vi "RSxxx Protocol FG.vi"(7 "Action":T1, 8 "error in (no error)":errorcluster, 10 "Serial Config":T2={"Port"="COM1", "Baud Rate"=9600, "Data Bits"=8, "Parity"=enum."None", "Stop Bits"=10, "Flow Control"=0, "XON"=enum."DC1", "XOFF"=enum."DC3", "End Read on Termination Character"=TRUE, "End Write on Termination Character"=TRUE, "Termination Character"=10} {"Termination Character" format="%.0x"; "Flow Control" items=["None"=0, "XON/XOFF"=1, "RTS/CTS"=2, "DTR/DSR"=4]; "Stop Bits" items=["1.0"=10, "1.5"=15, "2.0"=20]; "Data Bits" min=5 max=8 step=1; "Baud Rate" items=["75"=75, "110"=110, "134"=134, "150"=150, "300"=300, "600"=600, "1200"=1200, "1800"=1800, "2400"=2400, "4800"=4800, "7200"=7200, "9600"=9600, "14400"=14400, "19200"=19200, "28800"=28800, "38400"=38400, "56000"=56000, "57600"=57600, "115200"=115200, "128000"=128000, "230400"=230400, "460800"=460800, "921600"=921600, "1843200"=1843200, "3000000"=3000000]}, 11 "Device Item Ref in":T3 format="%.0x") -> (0 "error out":errorcluster, 2 "Serial Config":T2 {"Termination Character" format="%.0x"; "Flow Control" items=["None"=0, "XON/XOFF"=1, "RTS/CTS"=2, "DTR/DSR"=4]; "Stop Bits" items=["1.0"=10, "1.5"=15, "2.0"=20]; "Data Bits" min=5 max=8 step=1; "Baud Rate" items=["75"=75, "110"=110, "134"=134, "150"=150, "300"=300, "600"=600, "1200"=1200, "1800"=1800, "2400"=2400, "4800"=4800, "7200"=7200, "9600"=9600, "14400"=14400, "19200"=19200, "28800"=28800, "38400"=38400, "56000"=56000, "57600"=57600, "115200"=115200, "128000"=128000, "230400"=230400, "460800"=460800, "921600"=921600, "1843200"=1843200, "3000000"=3000000]}, 3 "Item Ref out":T3 format="%.0x")   [LabVIEW 2018, in "Instrument Addon Shared.lvlib"]
uses:
  Instrument Addon Shared.lvlib
  <vilib>/NI Veristand/Custom Device API/Custom Device Item Ref.ctl
  Types/RSXXX Port Settings.ctl
  Types/FG Control.ctl
  Constants.vi
  <vilib>/NI Veristand/Custom Device API/Get Item Property (String).vi
  <vilib>/NI Veristand/Custom Device API/Get Item Property (U32).vi
  <vilib>/NI Veristand/Custom Device API/Get Item Property (Boolean).vi
  <vilib>/NI Veristand/Custom Device API/Set Item Property (String).vi
  <vilib>/NI Veristand/Custom Device API/Set Item Property (U32).vi
  <vilib>/NI Veristand/Custom Device API/Set Item Property (Boolean).vi
  <vilib>/NI Veristand/Custom Device API/Custom Device API.lvlib
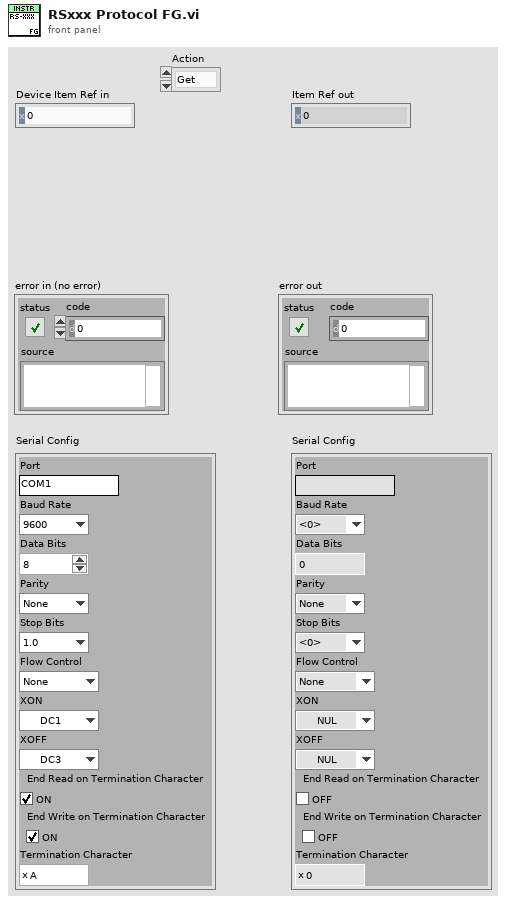
[diagram p1: front panel]
types:
  T1 = typedef "Instrument Addon Shared.lvlib/FG Control.ctl" = enum16{"Get", "Set"}
  T2 = typedef "Instrument Addon Shared.lvlib/RSXXX Port Settings.ctl" = cluster{"Port":string, "Baud Rate":u32, "Data Bits":u16, "Parity":enum16{"None", "Odd", "Even", "Mark", "Space"}, "Stop Bits":u16, "Flow Control":u16, "XON":enum16{"NUL", "SOH", "STX", "ETX", "EOT", "ENQ", "ACK", "BEL", "BS", "HT", "LF", "VT", "FF", "CR", "SO", "SI", "DLE", "DC1", "DC2", "DC3", "DC4", "NAK", "SYN", "ETB", "CAN", "EM", "SUB", "ESC", "FS", "GS", "RS", "US", "SP", "!", "\"", "#", "$", "%", "&", "'", "(", ")", "*", "+", ",", "- (-)", ".", "/", "0", "1", "2", "3", "4", "5", "6", "7", "8", "9", ":", ";", "<", "=", ">", "?", "@", "A", "B", "C", "D", "E", "F", "G", "H", "I", "J", "K", "L", "M", "N", "O", "P", "Q", "R", "S", "T", "U", "V", "W", "X", "Y", "Z", "[", "\\", "]", "^", "_", "`", "a", "b", "c", "d", "e", "f", "g", "h", "i", "j", "k", "l", "m", "n", "o", "p", "q", "r", "s", "t", "u", "v", "w", "x", "y", "z", "{", "|", "}", "~"}, "XOFF":enum16{"NUL", "SOH", "STX", "ETX", "EOT", "ENQ", "ACK", "BEL", "BS", "HT", "LF", "VT", "FF", "CR", "SO", "SI", "DLE", "DC1", "DC2", "DC3", "DC4", "NAK", "SYN", "ETB", "CAN", "EM", "SUB", "ESC", "FS", "GS", "RS", "US", "SP", "!", "\"", "#", "$", "%", "&", "'", "(", ")", "*", "+", ",", "- (-)", ".", "/", "0", "1", "2", "3", "4", "5", "6", "7", "8", "9", ":", ";", "<", "=", ">", "?", "@", "A", "B", "C", "D", "E", "F", "G", "H", "I", "J", "K", "L", "M", "N", "O", "P", "Q", "R", "S", "T", "U", "V", "W", "X", "Y", "Z", "[", "\\", "]", "^", "_", "`", "a", "b", "c", "d", "e", "f", "g", "h", "i", "j", "k", "l", "m", "n", "o", "p", "q", "r", "s", "t", "u", "v", "w", "x", "y", "z", "{", "|", "}", "~"}, "End Read on Termination Character":bool, "End Write on Termination Character":bool, "Termination Character":u8}
  T3 = typedef "Custom Device API.lvlib/Custom Device Item Ref.ctl" = u64
  T4 = enum16{"NUL", "SOH", "STX", "ETX", "EOT", "ENQ", "ACK", "BEL", "BS", "HT", "LF", "VT", "FF", "CR", "SO", "SI", "DLE", "DC1", "DC2", "DC3", "DC4", "NAK", "SYN", "ETB", "CAN", "EM", "SUB", "ESC", "FS", "GS", "RS", "US", "SP", "!", "\"", "#", "$", "%", "&", "'", "(", ")", "*", "+", ",", "- (-)", ".", "/", "0", "1", "2", "3", "4", "5", "6", "7", "8", "9", ":", ";", "<", "=", ">", "?", "@", "A", "B", "C", "D", "E", "F", "G", "H", "I", "J", "K", "L", "M", "N", "O", "P", "Q", "R", "S", "T", "U", "V", "W", "X", "Y", "Z", "[", "\\", "]", "^", "_", "`", "a", "b", "c", "d", "e", "f", "g", "h", "i", "j", "k", "l", "m", "n", "o", "p", "q", "r", "s", "t", "u", "v", "w", "x", "y", "z", "{", "|", "}", "~"}
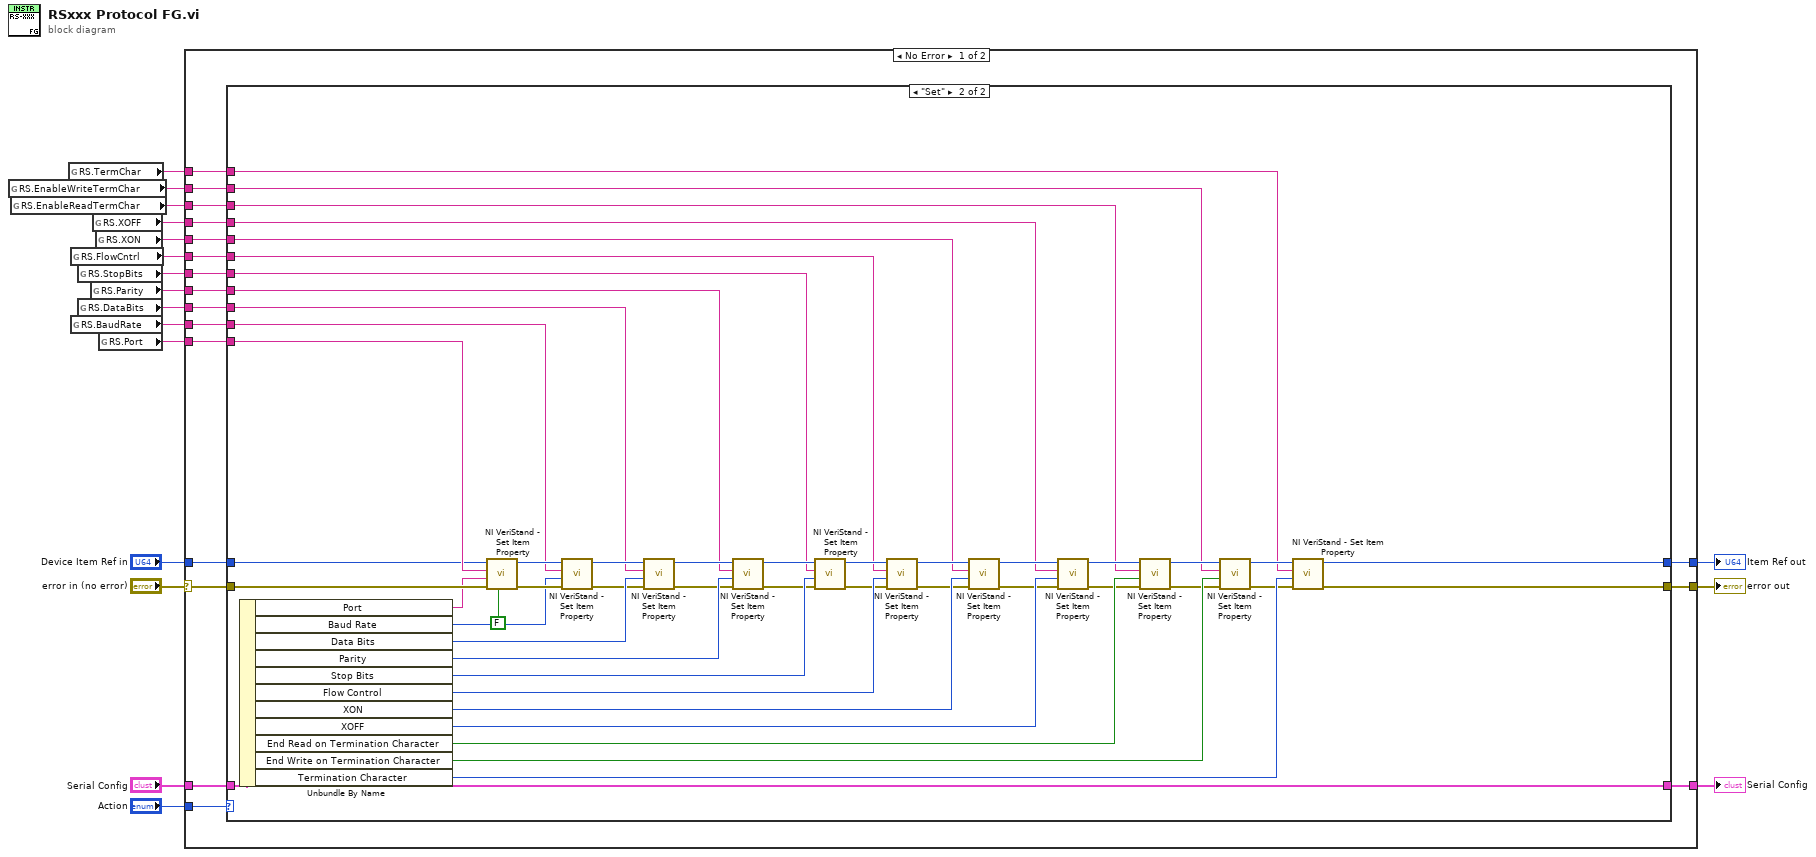
[diagram p0: block diagram]
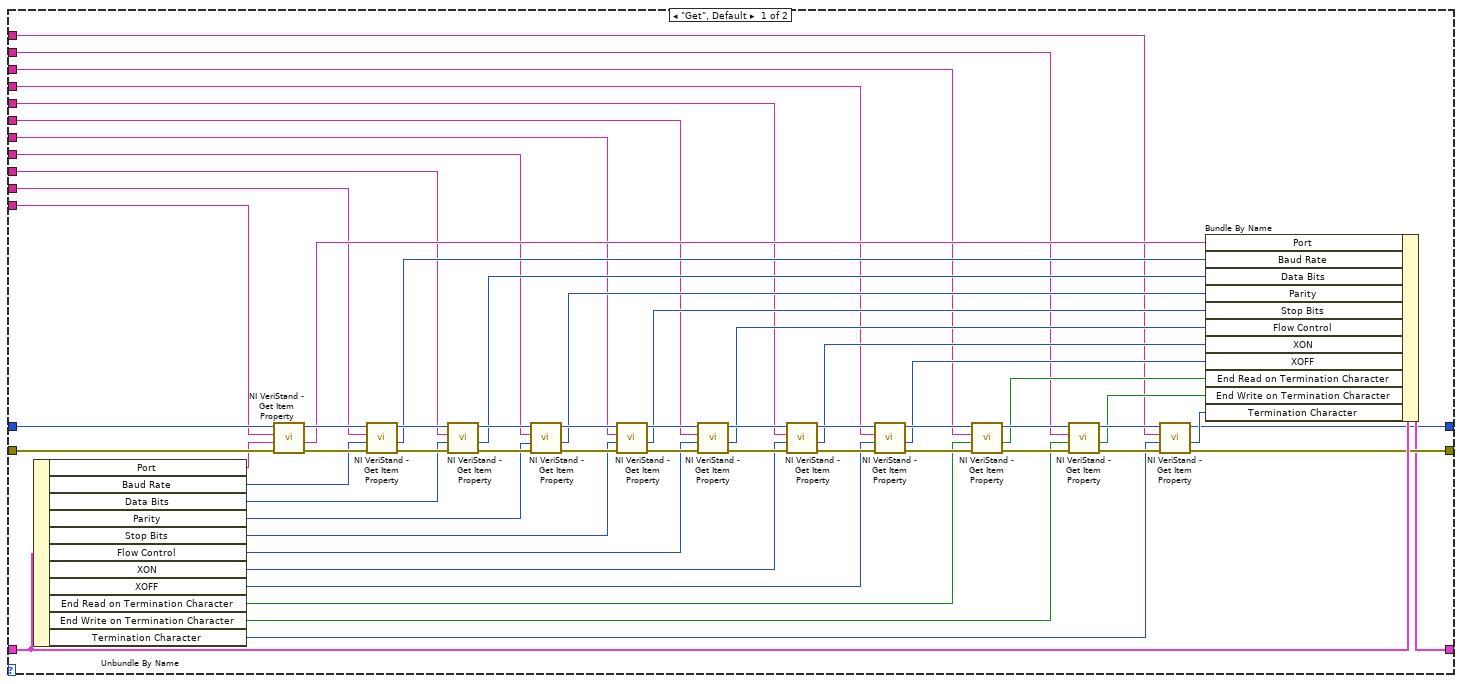
[diagram p2: hidden frame]
diagram:
  n1 = global read "Constants.vi" "RS.EnableWriteTermChar"() -> (w2:string)
  n2 = global read "Constants.vi" "RS.EnableReadTermChar"() -> (w3:string)
  n3 = global read "Constants.vi" "RS.TermChar"() -> (w1:string)
  n4 = global read "Constants.vi" "RS.FlowCntrl"() -> (w6:string)
  n5 = global read "Constants.vi" "RS.BaudRate"() -> (w10:string)
  n6 = global read "Constants.vi" "RS.StopBits"() -> (w7:string)
  n7 = global read "Constants.vi" "RS.DataBits"() -> (w9:string)
  n8 = global read "Constants.vi" "RS.Parity"() -> (w8:string)
  n9 = global read "Constants.vi" "RS.XOFF"() -> (w4:string)
  n10 = global read "Constants.vi" "RS.XON"() -> (w5:string)
  n11 = global read "Constants.vi" "RS.Port"() -> (w18:string)
  n12 = case shown="No Error" "error in (no error)" {
    selector: "error in (no error)" -> [w31 w146]
    tunnel: w18 -> [w36 _]
    tunnel: [w35 w144] -> w17
    tunnel: "Device Item Ref in" -> [w34 w144]
    tunnel: "Serial Config" -> [w33 w145]
    tunnel: [w32 w146] -> w14
    tunnel: [w30 w145] -> w12
    tunnel: "Action" -> [w29 _]
    tunnel: w10 -> [w28 _]
    tunnel: w9 -> [w27 _]
    tunnel: w8 -> [w26 _]
    tunnel: w7 -> [w25 _]
    tunnel: w6 -> [w24 _]
    tunnel: w5 -> [w23 _]
    tunnel: w4 -> [w22 _]
    tunnel: w3 -> [w21 _]
    tunnel: w2 -> [w20 _]
    tunnel: w1 -> [w19 _]
    frame No Error {
      n13 = case shown="\"Set\"" w29 {
        tunnel: w36 -> [w93 w143]
        tunnel: [w47 w106] -> w35
        tunnel: w34 -> [w94 w142]
        tunnel: w33 -> [w61 w140]
        tunnel: [w49 w107] -> w32
        tunnel: w31 -> [w95 w141]
        tunnel: [w48 w140] -> w30
        tunnel: w28 -> [w46 w105]
        tunnel: w27 -> [w45 w104]
        tunnel: w26 -> [w44 w103]
        tunnel: w25 -> [w43 w102]
        tunnel: w24 -> [w42 w101]
        tunnel: w23 -> [w41 w100]
        tunnel: w22 -> [w40 w99]
        tunnel: w21 -> [w39 w98]
        tunnel: w20 -> [w38 w97]
        tunnel: w19 -> [w37 w96]
        frame "Get", Default {
          n14 = Unbundle By Name(w61) -> ("Port"=w92:string, "Baud Rate"=w71:u32, "Data Bits"=w70:u16, "Parity"=w69:enum16{"None", "Odd", "Even", "Mark", "Space"}, "Stop Bits"=w68:u16, "Flow Control"=w67:u16, "XON"=w66:T4, "XOFF"=w65:T4, "End Read on Termination Character"=w64:bool, "End Write on Termination Character"=w63:bool, "Termination Character"=w62:u8)
          n15 = call-poly <vilib>:"NI VeriStand - Get Item Property.vi"("error in (no error)"=w95, "Default Value"=w92, "Property Name"=w93, "Item Ref in"=w94) -> ("error out"=w81:errorcluster, "Value"=w60:string, "Item Ref out"=w91:T3)  [unwired: 4 in, 1 out]
          n16 = call-poly <vilib>:"NI VeriStand - Get Item Property.vi"("error in (no error)"=w81, "Default Value"=w71, "Property Name"=w46, "Item Ref in"=w91) -> ("error out"=w80:errorcluster, "Value"=w59:u32, "Item Ref out"=w90:T3)  [unwired: 4 in, 1 out]
          n17 = call-poly <vilib>:"NI VeriStand - Get Item Property.vi"("error in (no error)"=w80, "Default Value"=w70, "Property Name"=w45, "Item Ref in"=w90) -> ("error out"=w79:errorcluster, "Value"=w58:u32, "Item Ref out"=w89:T3)  [unwired: 4 in, 1 out]
          n18 = call-poly <vilib>:"NI VeriStand - Get Item Property.vi"("error in (no error)"=w79, "Default Value"=w69, "Property Name"=w44, "Item Ref in"=w89) -> ("error out"=w78:errorcluster, "Value"=w57:u32, "Item Ref out"=w88:T3)  [unwired: 4 in, 1 out]
          n19 = call-poly <vilib>:"NI VeriStand - Get Item Property.vi"("error in (no error)"=w78, "Default Value"=w68, "Property Name"=w43, "Item Ref in"=w88) -> ("error out"=w77:errorcluster, "Value"=w56:u32, "Item Ref out"=w87:T3)  [unwired: 4 in, 1 out]
          n20 = call-poly <vilib>:"NI VeriStand - Get Item Property.vi"("error in (no error)"=w77, "Default Value"=w67, "Property Name"=w42, "Item Ref in"=w87) -> ("error out"=w76:errorcluster, "Value"=w55:u32, "Item Ref out"=w86:T3)  [unwired: 4 in, 1 out]
          n21 = call-poly <vilib>:"NI VeriStand - Get Item Property.vi"("error in (no error)"=w76, "Default Value"=w66, "Property Name"=w41, "Item Ref in"=w86) -> ("error out"=w75:errorcluster, "Value"=w54:u32, "Item Ref out"=w85:T3)  [unwired: 4 in, 1 out]
          n22 = call-poly <vilib>:"NI VeriStand - Get Item Property.vi"("error in (no error)"=w75, "Default Value"=w65, "Property Name"=w40, "Item Ref in"=w85) -> ("error out"=w74:errorcluster, "Value"=w53:u32, "Item Ref out"=w84:T3)  [unwired: 4 in, 1 out]
          n23 = call-poly <vilib>:"NI VeriStand - Get Item Property.vi"("error in (no error)"=w74, "Default Value"=w64, "Property Name"=w39, "Item Ref in"=w84) -> ("error out"=w73:errorcluster, "Value"=w52:bool, "Item Ref out"=w83:T3)  [unwired: 4 in, 1 out]
          n24 = call-poly <vilib>:"NI VeriStand - Get Item Property.vi"("error in (no error)"=w73, "Default Value"=w63, "Property Name"=w38, "Item Ref in"=w83) -> ("error out"=w72:errorcluster, "Value"=w51:bool, "Item Ref out"=w82:T3)  [unwired: 4 in, 1 out]
          n25 = call-poly <vilib>:"NI VeriStand - Get Item Property.vi"("error in (no error)"=w72, "Default Value"=w62, "Property Name"=w37, "Item Ref in"=w82) -> ("error out"=w49:errorcluster, "Value"=w50:u32, "Item Ref out"=w47:T3)  [unwired: 4 in, 1 out]
          n26 = Bundle By Name(cluster=w61, "Port"=w60, "Baud Rate"=w59, "Data Bits"=w58, "Parity"=w57, "Stop Bits"=w56, "Flow Control"=w55, "XON"=w54, "XOFF"=w53, "End Read on Termination Character"=w52, "End Write on Termination Character"=w51, "Termination Character"=w50) -> (w48:T2)
        }
        frame "Set" {
          n27 = Unbundle By Name(w140) -> ("Port"=w139:string, "Baud Rate"=w136:u32, "Data Bits"=w134:u16, "Parity"=w133:enum16{"None", "Odd", "Even", "Mark", "Space"}, "Stop Bits"=w132:u16, "Flow Control"=w131:u16, "XON"=w130:T4, "XOFF"=w129:T4, "End Read on Termination Character"=w128:bool, "End Write on Termination Character"=w127:bool, "Termination Character"=w126:u8)
          n28 = call-poly <vilib>:"NI VeriStand - Set Item Property.vi"("Binary String (T)"=FALSE, "error in (no error)"=w141, "Value"=w139, "Property Name"=w143, "Item Ref in"=w142) -> ("error out"=w137:errorcluster, "Item Ref out"=w135:T3)  [unwired: 4 in, 1 out]
          n29 = call-poly <vilib>:"NI VeriStand - Set Item Property.vi"("error in (no error)"=w137, "Value"=w136, "Property Name"=w105, "Item Ref in"=w135) -> ("error out"=w125:errorcluster, "Item Ref out"=w116:T3)  [unwired: 5 in, 1 out]
          n30 = call-poly <vilib>:"NI VeriStand - Set Item Property.vi"("error in (no error)"=w125, "Value"=w134, "Property Name"=w104, "Item Ref in"=w116) -> ("error out"=w124:errorcluster, "Item Ref out"=w115:T3)  [unwired: 5 in, 1 out]
          n31 = call-poly <vilib>:"NI VeriStand - Set Item Property.vi"("error in (no error)"=w124, "Value"=w133, "Property Name"=w103, "Item Ref in"=w115) -> ("error out"=w123:errorcluster, "Item Ref out"=w114:T3)  [unwired: 5 in, 1 out]
          n32 = call-poly <vilib>:"NI VeriStand - Set Item Property.vi"("error in (no error)"=w123, "Value"=w132, "Property Name"=w102, "Item Ref in"=w114) -> ("error out"=w122:errorcluster, "Item Ref out"=w113:T3)  [unwired: 5 in, 1 out]
          n33 = call-poly <vilib>:"NI VeriStand - Set Item Property.vi"("error in (no error)"=w122, "Value"=w131, "Property Name"=w101, "Item Ref in"=w113) -> ("error out"=w121:errorcluster, "Item Ref out"=w112:T3)  [unwired: 5 in, 1 out]
          n34 = call-poly <vilib>:"NI VeriStand - Set Item Property.vi"("error in (no error)"=w121, "Value"=w130, "Property Name"=w100, "Item Ref in"=w112) -> ("error out"=w120:errorcluster, "Item Ref out"=w111:T3)  [unwired: 5 in, 1 out]
          n35 = call-poly <vilib>:"NI VeriStand - Set Item Property.vi"("error in (no error)"=w120, "Value"=w129, "Property Name"=w99, "Item Ref in"=w111) -> ("error out"=w119:errorcluster, "Item Ref out"=w110:T3)  [unwired: 5 in, 1 out]
          n36 = call-poly <vilib>:"NI VeriStand - Set Item Property.vi"("error in (no error)"=w119, "Value"=w128, "Property Name"=w98, "Item Ref in"=w110) -> ("error out"=w118:errorcluster, "Item Ref out"=w109:T3)  [unwired: 5 in, 1 out]
          n37 = call-poly <vilib>:"NI VeriStand - Set Item Property.vi"("error in (no error)"=w118, "Value"=w127, "Property Name"=w97, "Item Ref in"=w109) -> ("error out"=w117:errorcluster, "Item Ref out"=w108:T3)  [unwired: 5 in, 1 out]
          n38 = call-poly <vilib>:"NI VeriStand - Set Item Property.vi"("error in (no error)"=w117, "Value"=w126, "Property Name"=w96, "Item Ref in"=w108) -> ("error out"=w107:errorcluster, "Item Ref out"=w106:T3)  [unwired: 5 in, 1 out]
        }
      }
    }
    frame Error {
    }
  }
  "Item Ref out" <- w17
  "error out" <- w14
  "Serial Config" <- w12
